vi "MM6.PG_MultiplyMultiplePattern_SuperHyperKnorz.vi"(0 "i ref in":refnum<vi>, 2 "PGDataType":T1, 5 "error in (no error)":errorcluster) -> (14 "i ref out":refnum<vi>, 16 "PGData":T1, 19 "error out":errorcluster)   [LabVIEW 2014, in "MM6.lvlib"]
doc: "This vi manipulates the PG data to repeat a pattern datum several times."
uses:
  MM6.lvlib
  CSDigitalIO/PPG_ABC/PPG_ABC.PG_dataType.ctl
  CSDigitalIO/PPG_ABC/PPG_ABC.lvlib
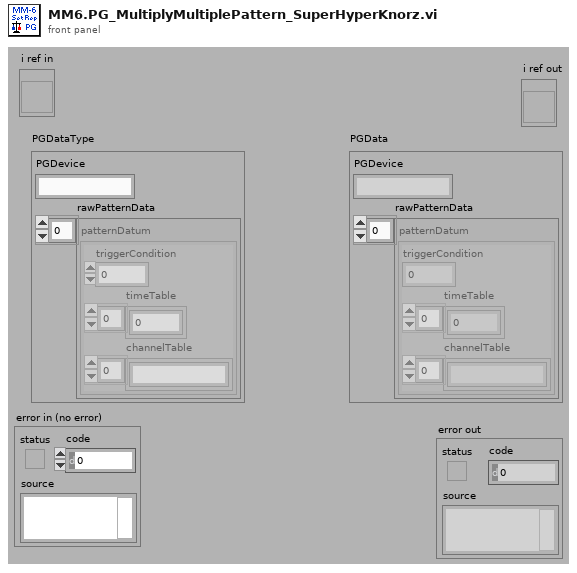
[diagram p1: front panel]
types:
  T1 = typedef "PPG_ABC.lvlib/PPG_ABC.PG_dataType.ctl" = cluster{"PGDevice":string, "rawPatternData":cluster{"triggerCondition":i32, "timeTable":dbl[], "channelTable":string[]}[]}
  T2 = typedef "MM6.lvlib/MM6.i attribute.ctl" = cluster{"ConfigData":T3, "UsedObjs":string[], "ActScanStep":i32[], "AbortRequest":bool, "StopRequest":bool, "# cycles":i32, "Connected":bool, "MMStatus":T18, "# data":i32, "DIMServices":cluster{"MM6StatusString":string, "MM6StatusID":i32, "discArchiver":string, "discArchiverID":i32, "eventBuilder":string, "eventBuilderID":i32, "GUIIDString":string, "GUIIDStringID":i32}, "dataFile":string, "ExtraDataSets":T19, "PGRunning":T20}
  T3 = typedef "LEBITDefs.lvlib/LEBITDefs.ConfigData.ctl" = cluster{"GenConfig":T4, "Configs":T6[]}
  T4 = typedef "LEBITDefs.lvlib/LEBITDefs.GenConfig.ctl" = cluster{"Mode":i32, "Logs":T5[]}
  T5 = typedef "LEBITDefs.lvlib/LEBITDefs.Log.ctl" = cluster{"Name":string, "FctName":string, "Special":string}
  T6 = typedef "LEBITDefs.lvlib/LEBITDefs.OneConfig.ctl" = cluster{"MCA":T7, "Timing":T8, "Scans":T11[], "FreqDevs":T12[], "CleanDev":T13, "NrCycles":i32, "Specials":T15[], "Delays":T16[], "DAC":T17}
  T7 = typedef "LEBITDefs.lvlib/LEBITDefs.MCA.ctl" = cluster{"Name":string, "Address":string, "NrChannels":i32, "Gate":i32, "NrPipse":i32}
  T8 = typedef "LEBITDefs.lvlib/LEBITDefs.Timing.ctl" = cluster{"TimeTables":cluster{"TimeTable":T9}[], "Memories":T10[], "ScanX":string, "ScanY":string}
  T9 = typedef "LEBITDefs.lvlib/LEBITDefs.Timetable.ctl" = dbl[]
  T10 = typedef "LEBITDefs.lvlib/LEBITDefs.Memory.ctl" = cluster{"Device":string, "ExtTrig":bool, "TT2Use":i32, "PatternTable":string[]}
  T11 = typedef "LEBITDefs.lvlib/LEBITDefs.ScanDev.ctl" = cluster{"Name":string, "FctName":string, "Values":dbl[], "NrScanVals":i32, "Special":string}
  T12 = typedef "LEBITDefs.lvlib/LEBITDefs.FreqDev.ctl" = cluster{"Name":string, "Amp":dbl, "CenterFreq":dbl, "Time":dbl}
  T13 = typedef "LEBITDefs.lvlib/LEBITDefs.CleanDev.ctl" = cluster{"Name":string, "CleanData":T14[]}
  T14 = typedef "LEBITDefs.lvlib/LEBITDefs.CleanDataType.ctl" = cluster{"Amp":dbl, "Center":dbl, "Plus":dbl, "Minus":dbl, "Time":dbl}
  T15 = typedef "LEBITDefs.lvlib/LEBITDefs.Special.ctl" = cluster{"Name":string, "FctName":string, "VerySpecial":string, "Data":dbl}
  T16 = typedef "LEBITDefs.lvlib/LEBITDefs.Delay.ctl" = cluster{"Name":string, "Delay":dbl}
  T17 = typedef "LEBITDefs.lvlib/LEBITDefs.DAC.ctl" = cluster{"Name":string, "Step1":i32, "Step2":i32}
  T18 = typedef "MM6.lvlib/MM6.status.ctl" = enum16{"loaded", "load_error", "config", "config_error", "init", "init_error", "data_reset", "data_reset_error", "running", "start_error", "run_error", "abort_requested", "aborted", "stop_requested", "stopped", "stop_error", "Connected", "NOTConnected"}
  T19 = typedef "LEBITDefs.lvlib/LEBITDefs.ExtraData.ctl" = cluster{"Ions":cluster{"ExcitIonMass":string, "ExcitIonCharge":i32, "CleanIons":cluster{"CleanIonMass":string, "CleanIonCharge":i32}[]}, "TimingDescription":cluster{"TimeTableDescription":cluster{"Times":string[]}[], "PatternTableDescription":cluster{"Pattern":string[]}[]}, "ScanUnits":string[]}[]
  T20 = typedef "PPG_ABC.lvlib/PPG_ABC.PG_Running.ctl" = i32
  T21 = typedef "MM6.lvlib/MM6.MatchRepPattern.ctl" = enum16{"noMatch", "oneTG", "twoTG"}
  T22 = cluster{"triggerCondition":i32, "timeTable":dbl[], "channelTable":string[]}[]
  T23 = cluster{"triggerCondition":i32, "timeTable":dbl[], "channelTable":string[]}
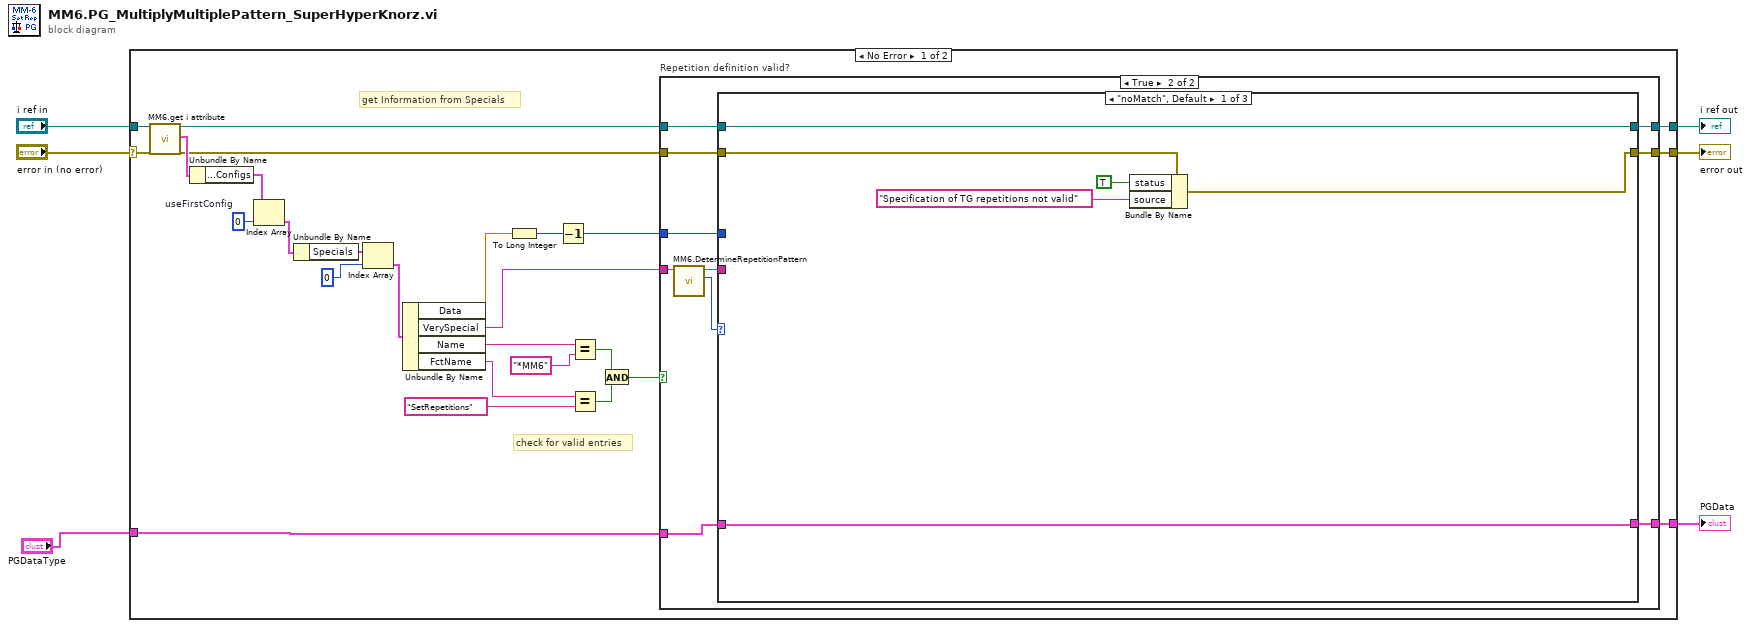
[diagram p0: block diagram]
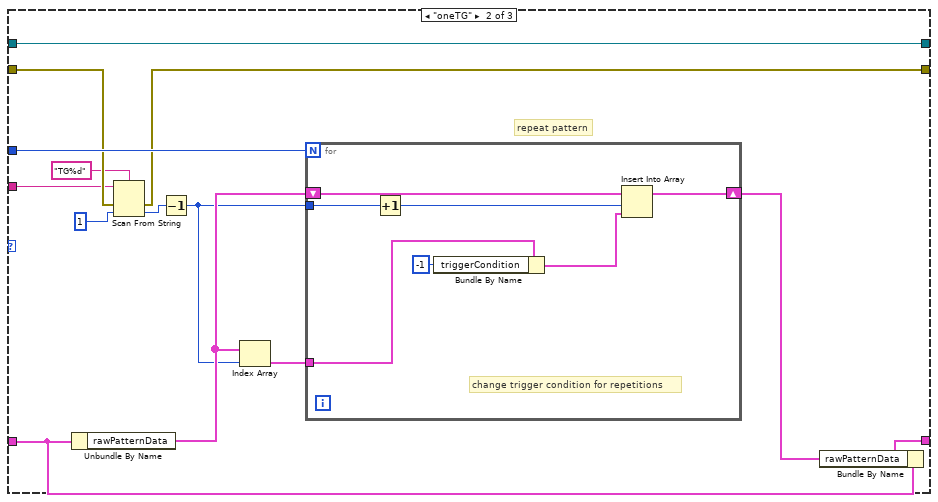
[diagram p3: hidden frame]
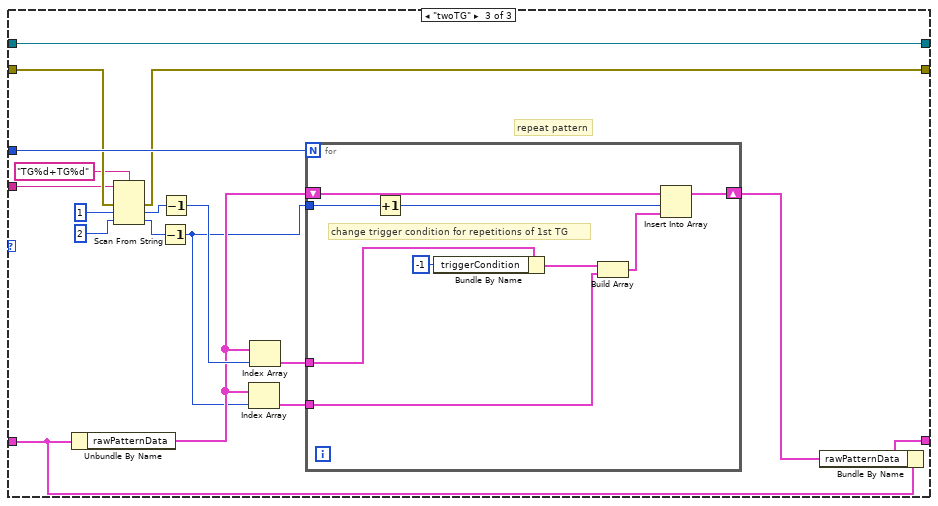
[diagram p4: hidden frame]
diagram:
  n1 = case shown="No Error" "error in (no error)" {
    selector: "error in (no error)" -> [w14 w101]
    tunnel: "i ref in" -> [w15 w102]
    tunnel: [w26 w102] -> w5
    tunnel: [w25 w101] -> w4
    tunnel: "PGDataType" -> [w16 w100]
    tunnel: [w17 w100] -> w1
    frame No Error {
      w30 = 0  # useFirstConfig
      # "check for valid entries"
      # "get Information from Specials"
      n2 = call "MM6.get i attribute.vi"("i ref in"=w15, "error in (no error)"=w14) -> ("i ref out"=w28:refnum<vi>, "i attribute"=w32:T2, "error out"=w27:errorcluster)  [unwired: 15 in]
      n3 = Unbundle By Name(w32) -> ("ConfigData.Configs"=w31:T6[])
      n4 = Index Array(array=w31, index=w30) -> (element=w29:T6)
      n5 = Unbundle By Name(w29) -> ("Specials"=w24:T15[])
      n6 = Index Array(array=w24, index=0) -> (element=w22:T15)
      n7 = Unbundle By Name(w22) -> ("Data"=w10:dbl, "VerySpecial"=w7:string, "Name"=w9:string, "FctName"=w8:string)
      n8 = To Long Integer(number=w10) -> (32bit integer=w12:i32)
      n9 = Decrement(x=w12) -> (x-1=w11:i32)
      n10 = Equal?(x=w9, y="*MM6") -> (x = y?=w19:bool)
      n11 = Equal?(x=w8, y="SetRepetitions") -> (x = y?=w18:bool)
      n12 = And(x=w19, y=w18) -> (x .and. y?=w13:bool)
      n13 = case "Repetition definition valid?" shown="True" w13 {
        tunnel: w28 -> [w35 w42]
        tunnel: w27 -> [w34 w41]
        tunnel: [w35 w39] -> w26
        tunnel: [w34 w40] -> w25
        tunnel: w11 -> [_ w43]
        tunnel: [w33 w45] -> w17
        tunnel: w16 -> [w33 w44]
        tunnel: w7 -> [_ w38]
        frame False {
        }
        frame True {
          n14 = call "MM6.DetermineRepetitionPattern.vi"("string"=w38) -> ("MatchPattern"=w36:T21, "string out"=w37:string)  [unwired: 9 in]
          n15 = case shown="\"noMatch\", Default" w36 {
            tunnel: [w50 w65 w90] -> w45
            tunnel: w44 -> [w50 w64 w89]
            tunnel: w43 -> [_ w60 w86]
            tunnel: w37 -> [_ w54 w80]
            tunnel: w42 -> [w51 w58 w84]
            tunnel: w41 -> [w48 w57 w83]
            tunnel: [w49 w56 w82] -> w40
            tunnel: [w51 w58 w84] -> w39
            frame "noMatch", Default {
              n16 = Bundle By Name(cluster=w48, "status"=TRUE, "source"="Specification of TG repetitions not valid") -> (w49:errorcluster)
            }
            frame "oneTG" {
              # "repeat pattern"
              n17 = Unbundle By Name(w64) -> ("rawPatternData"=w62:T22)
              n18 = Scan From String(format string="TG%d", input string=w54, error in=w57, default 1=1) -> (error out=w56:errorcluster, output 1=w52:i32)  [unwired: 1 in, 2 out]
              n19 = Decrement(x=w52) -> (x-1=w59:i32)
              n20 = Index Array(array=w62, index=w59) -> (element=w61:T23)
              n21 = for {
                N: w60 -> [_]
                shift-right: [w72] -> w63
                shift-left: w62 -> [w71]
                tunnel: w59 -> [w70]
                tunnel: w61 -> [w66]
                # "change trigger condition for repetitions"
                n22 = Increment(x=w70) -> (x+1=w68:i32)
                n23 = Bundle By Name(cluster=w66, "triggerCondition"=-1) -> (w69:T23)
                n24 = Insert Into Array(array=w71, index=w68, new element=w69) -> (w72:T22)
              }
              n25 = Bundle By Name(cluster=w64, "rawPatternData"=w63) -> (w65:T1)
            }
            frame "twoTG" {
              # "repeat pattern"
              n26 = Unbundle By Name(w89) -> ("rawPatternData"=w75:T22)
              n27 = Scan From String(format string="TG%d+TG%d", input string=w80, error in=w83, default 1=1, default 2=2) -> (error out=w82:errorcluster, output 1=w78:i32, output 2=w76:i32)  [unwired: 1 in, 2 out]
              n28 = Decrement(x=w76) -> (x-1=w73:i32)
              n29 = Decrement(x=w78) -> (x-1=w85:i32)
              n30 = Index Array(array=w75, index=w73) -> (element=w74:T23)
              n31 = Index Array(array=w75, index=w85) -> (element=w87:T23)
              n32 = for {
                N: w86 -> [_]
                shift-right: [w95] -> w88
                shift-left: w75 -> [w99]
                tunnel: w73 -> [w98]
                tunnel: w87 -> [w93]
                tunnel: w74 -> [w94]
                # "change trigger condition for repetitions of 1st TG"
                n33 = Increment(x=w98) -> (x+1=w97:i32)
                n34 = Bundle By Name(cluster=w93, "triggerCondition"=-1) -> (w91:T23)
                n35 = Build Array(w91, w94) -> (w92:T22)
                n36 = Insert Into Array(array=w99, index=w97, new element=w92) -> (w95:T22)
              }
              n37 = Bundle By Name(cluster=w89, "rawPatternData"=w88) -> (w90:T1)
            }
          }
        }
      }
    }
    frame Error {
    }
  }
  "error out" <- w4
  "i ref out" <- w5
  "PGData" <- w1
